vi "MakeOccupancyGrid.vi"() -> (1 "RealWorld":i16[][](graph), 2 "Occupancy Grid":i16[][](array[numeric]))   [LabVIEW 2014]
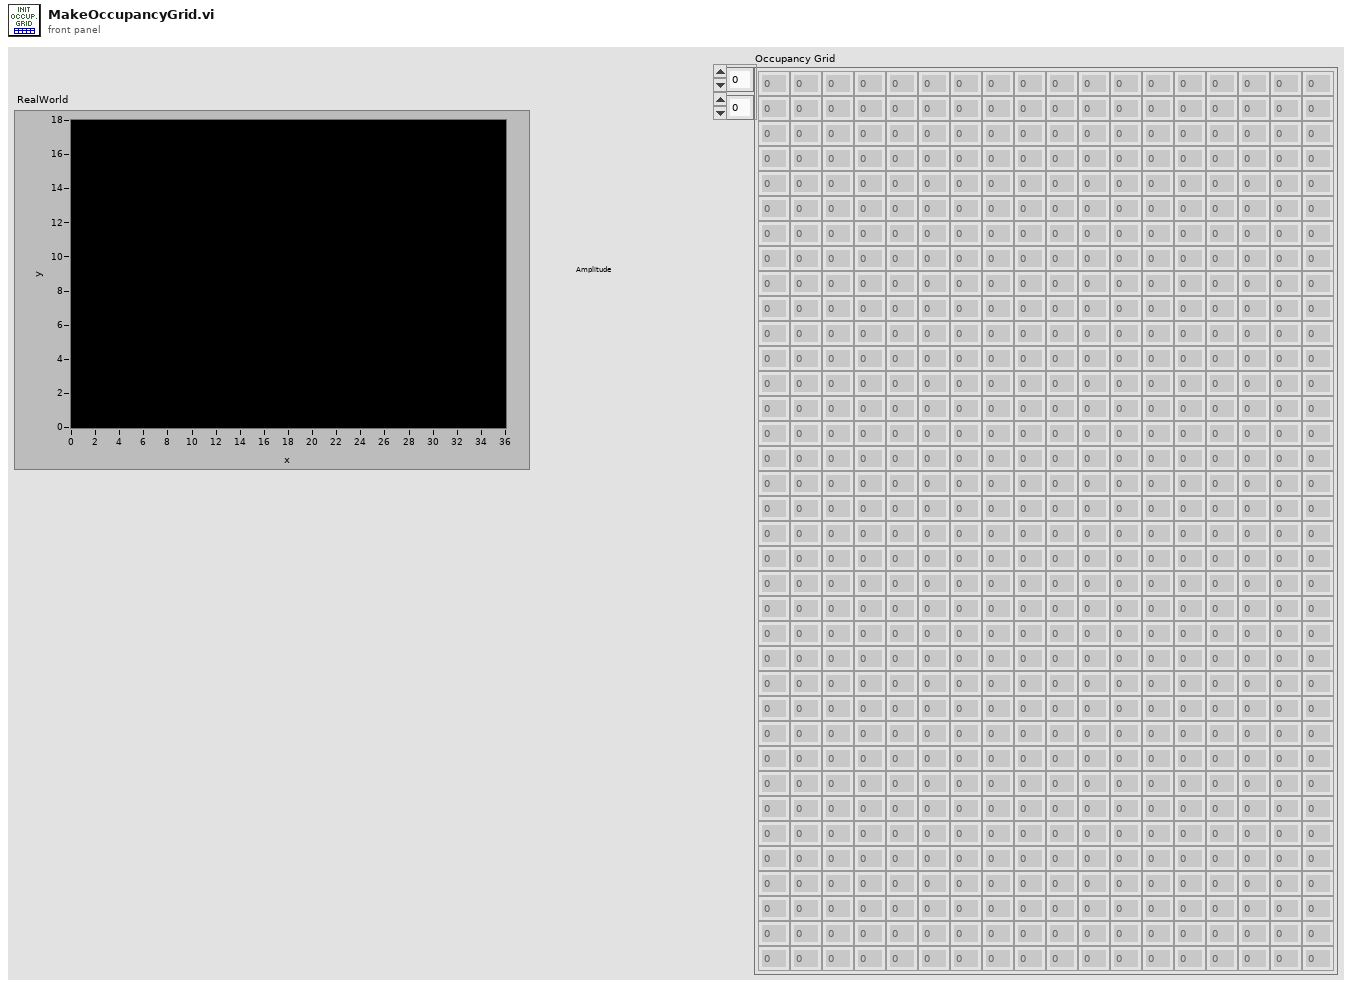
[diagram p1: front panel]
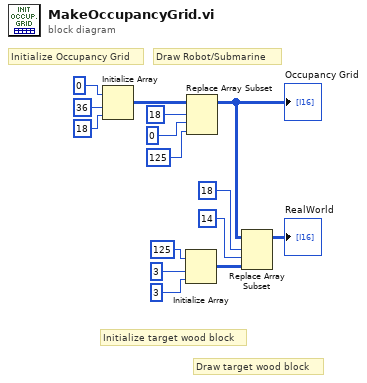
[diagram p0: block diagram]
diagram:
  # "Initialize target wood block"
  # "Draw target wood block"
  # "Draw Robot/Submarine"
  # "Initialize Occupancy Grid"
  n1 = Initialize Array(i16 0 ("element"), 36 ("dimension size"), 18 ("dimension size")) -> (w12:i16[][])
  n2 = Initialize Array(i16 125 ("element"), 3 ("dimension size"), 3 ("dimension size")) -> (w2:i16[][])
  n3 = Replace Array Subset(array=w12, new element=i16 125 ("new element/subarray"), index (row)=18, index (col)=0 ("disabled index (col)")) -> (w1:i16[][])
  "Occupancy Grid" <- w1
  n4 = Replace Array Subset(array=w1, new element=w2, index (row)=18, index (col)=14 ("disabled index (col)")) -> (→"RealWorld":i16[][])
